vi "Convert Transactions to String Arrays.vi"(8 "error in (no error)":errorcluster, 11 "Banking Statement in":refnum<class "Banking Statement.lvclass">) -> (0 "error out":errorcluster, 2 "String Arrays":string[](array[string]), 3 "Banking Statement out":refnum<class "Banking Statement.lvclass">)   [LabVIEW 2018, in "Banking Statement.lvclass"]
uses:
  Banking Statement.lvclass
  Banking Statement.lvclass/Banking Statement.ctl
  Banking Record/Banking Transaction.lvclass
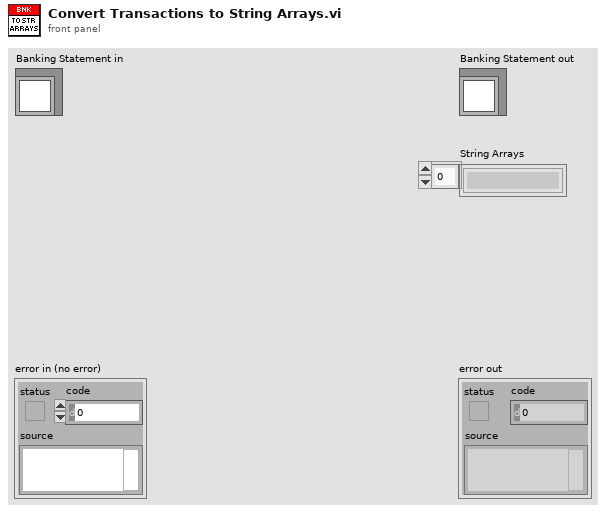
[diagram p1: front panel]
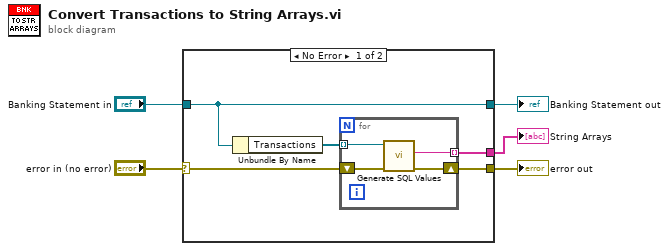
[diagram p0: block diagram]
diagram:
  n1 = case shown="No Error" "error in (no error)" {
    selector: "error in (no error)" -> [w8 w15]
    tunnel: "Banking Statement in" -> [w10 w16]
    tunnel: [w10 w16] -> w3
    tunnel: [w7 w15] -> w2
    tunnel: [w6 _] -> w1
    frame No Error {
      n2 = Unbundle By Name(w10) -> ("Transactions"=w9:refnum<class "Banking Transaction.lvclass">[])
      n3 = for {
        tunnel: w9 -> [w14] mode=indexing
        shift-right: [w12] -> w7
        shift-left: w8 -> [w13]
        tunnel: [w11] -> w6 mode=indexing
        n4 = call-dynamic "Generate SQL Values.vi"("error in (no error)"=w13, "Banking Record in"=w14) -> ("error out"=w12:errorcluster, "SQL Values"=w11:string)  [unwired: 7 in, 1 out]
      }
    }
    frame Error {
    }
  }
  "error out" <- w2
  "Banking Statement out" <- w3
  "String Arrays" <- w1
